vi "DrawDialog.vi"(8 "error in (no error)":errorcluster, 11 "Highscore in":refnum<class "HighscoreDialog.lvclass">) -> (0 "error out":errorcluster, 3 "Highscore out":refnum<class "HighscoreDialog.lvclass">)   [LabVIEW 2019, in "RT_Game.lvlib" / "HighscoreDialog.lvclass"]
uses:
  HighscoreDialog.lvclass
  C:/Users/FreshBob/Dropbox/VIs/myRIO_GameConsole/RT/RT_Game/GameObject/GameObject.lvclass
  Engine/Coordinate.ctl
  GameObject/GameObject.lvclass/GameObject.ctl
  HighscoreDialog.lvclass/HighscoreDialog.ctl
  GameObject/Read position.vi
  Engine/Engine.lvclass
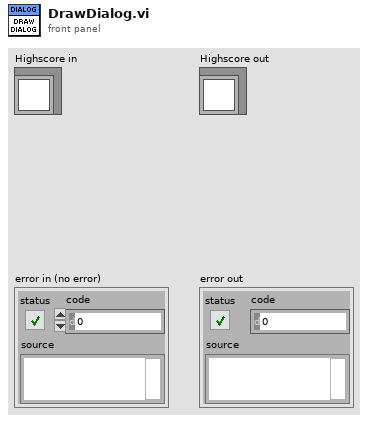
[diagram p1: front panel]
types:
  T1 = typedef "RT_Game.lvlib/Engine.lvclass/Coordinate.ctl" = cluster{"x":dbl, "y":dbl}
  T2 = typedef "RT_Game.lvlib/Game.lvclass/Coordinate.ctl" = cluster{"x":dbl, "y":dbl}
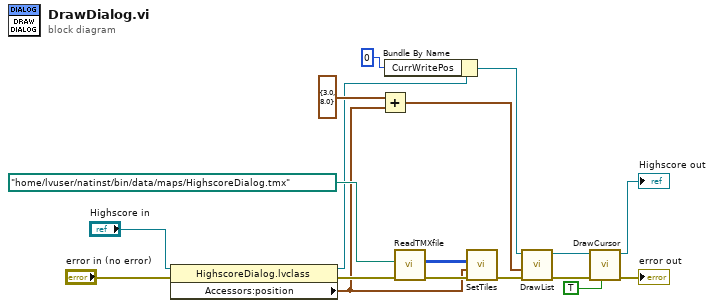
[diagram p0: block diagram]
diagram:
  n1 = property class="HighscoreDialog.lvclass"(reference="Highscore in", error in="error in (no error)") -> (reference out=w4:refnum<class "HighscoreDialog.lvclass">, error out=w6:errorcluster, "Accessors:position"=w1:T2)
  n2 = Add(x=T1 {"x"=3.0, "y"=8.0} ("y"), y=w1) -> (x+y=w16:T1)
  n3 = Bundle By Name(cluster=w4, "CurrWritePos"=i16 0 ("CurrPos")) -> (w3:refnum<class "HighscoreDialog.lvclass">)
  n4 = call "ReadTMXfile.vi"("error in (no error)"=w6, "path to tmx-file (created with Tiles2D)"=path "/home/lvuser/natinst/bin/data/maps/HighscoreDialog.tmx") -> ("error out"=w9:errorcluster, "Tilenumbers"=w12:u32[][])  [unwired: 8 in]
  n5 = call "SetTiles.vi"("error in (no error)"=w9, "Position"=w1, "TileCodes"=w12) -> ("error out"=w13:errorcluster)  [unwired: 8 in]
  n6 = call "DrawList.vi"("error in (no error)"=w13, "Position"=w16, "Highscore in"=w3) -> ("error out"=w14:errorcluster, "Highscore out"=w17:refnum<class "HighscoreDialog.lvclass">)  [unwired: 7 in]
  n7 = call "DrawCursor.vi"("Visible?"=TRUE, "error in (no error)"=w14, "Highscore in"=w17) -> ("error out"=→"error out":errorcluster, "Highscore out"=→"Highscore out":refnum<class "HighscoreDialog.lvclass">)  [unwired: 7 in]
